vi "plot_data_intermediateFill_Y.vi"(8 "plotData":i32[][](array[numeric]), 9 "idx Y (n)":i32, 10 "idx Y (n+1)":i32, 11 "idx X":i32) -> (0 "plotData out":i32[][](array[numeric]))   [LabVIEW 2010, in "OSA.lvclass"]
doc: "If difference in Y idx >1: fill intermidiate Y idx with 1."
uses:
  OSA.lvclass
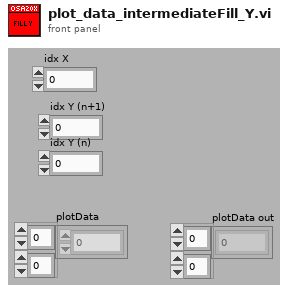
[diagram p1: front panel]
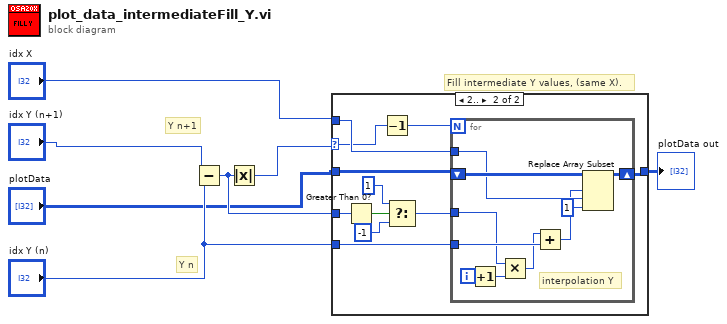
[diagram p0: block diagram]
diagram:
  # "Fill intermediate Y values, (same X)."
  # "Y n"
  # "Y n+1"
  n1 = Subtract(x="idx Y (n+1)", y="idx Y (n)") -> (x-y=w6:i32)
  n2 = Absolute Value(x=w6) -> (abs(x)=w7:i32)
  n3 = case shown="2.." w7 {
    selector: w7 -> [_ w10]
    tunnel: "plotData" -> [w8 w19]
    tunnel: [w8 w18] -> w1
    tunnel: "idx X" -> [_ w17]
    tunnel: "idx Y (n)" -> [_ w16]
    tunnel: w6 -> [_ w15]
    frame 0, Default {
    }
    frame 2.. {
      n4 = Greater Than 0?(x=w15) -> (x > 0?=w14:bool)
      n5 = Decrement(x=w10) -> (x-1=w9:i32)
      n6 = Select(t=1, s=w14, f=-1) -> (s? t:f=w11:i32)
      n7 = for {
        N: w9 -> [_]
        shift-right: [w28] -> w18
        shift-left: w19 -> [w29]
        tunnel: w17 -> [w27]
        tunnel: w16 -> [w26]
        tunnel: w11 -> [w25]
        i -> [w22]
        # "interpolation Y"
        n8 = Increment(x=w22) -> (x+1=w21:i32)
        n9 = Multiply(x=w25, y=w21) -> (x*y=w24:i32)
        n10 = Add(x=w24, y=w26) -> (x+y=w23:i32)
        n11 = Replace Array Subset(array=w29, new element=1 ("new element/subarray"), index (row)=w23, index (col)=w27) -> (w28:i32[][])
      }
    }
  }
  "plotData out" <- w1
